vi "globalSetUp.vi"(8 "error in (no error)":errorcluster, 11 "testcase-CSMWorkerMode.lvclass":refnum<class "testcase-CSMWorkerMode.lvclass">) -> (0 "error out":errorcluster, 3 "testcase-CSMWorkerMode.lvclass 2":refnum<class "testcase-CSMWorkerMode.lvclass">)   [LabVIEW 2017, in "testcase-CSMWorkerMode.lvclass"]
uses:
  testcase-CSMWorkerMode.lvclass
  <vilib>/addons/_JKI Toolkits/VI Tester/TestCase.llb/TestCase.lvclass
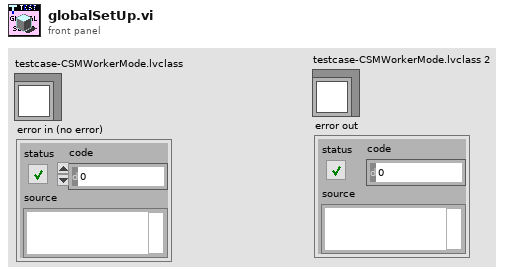
[diagram p1: front panel]
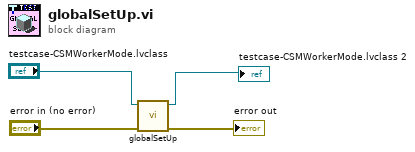
[diagram p0: block diagram]
diagram:
  n1 = call-parent "globalSetUp.vi"("error in (no error)"="error in (no error)", "TestCase in"="testcase-CSMWorkerMode.lvclass") -> ("error out"=→"error out":errorcluster, "TestCase out"=→"testcase-CSMWorkerMode.lvclass 2":refnum<class "testcase-CSMWorkerMode.lvclass">)  [unwired: 8 in]
